vi "libssh2_channel_subsystem.vi"(8 "error in (no error)":errorcluster, 10 "subsystem":string, 11 "channel":T1) -> (0 "error out":errorcluster)   [LabVIEW 2013, in "libssh2.lvlib"]
doc: "Initiates an subsystem-request on a session type channel."
uses:
  libssh2.lvlib
  Channel Refnum.ctl
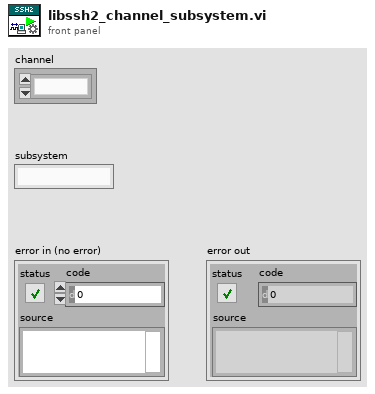
[diagram p1: front panel]
types:
  T1 = typedef "libssh2.lvlib/Channel Refnum.ctl" = refnum<k1>
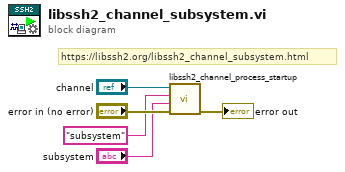
[diagram p0: block diagram]
diagram:
  # "https://libssh2.org/libssh2_channel_subsystem.html"
  n1 = call "libssh2_channel_process_startup.vi"("error in (no error)"="error in (no error)", "message"="subsystem", "request"="subsystem", "channel"="channel") -> ("error out"=→"error out":errorcluster)  [unwired: 7 in]
